vi "Update BrowerTree Component.vi"(6 "SymbolIndex":T1=enum."Project", 8 "error in (no error)":errorcluster, 9 "BrowerComponentNewName(\"\")":string, 10 "BrowerComponentID(\"\")":string, 11 "BrowerTree in":refnum<class "BrowerTree.lvclass">) -> (0 "error out":errorcluster, 3 "BrowerTree out":refnum<class "BrowerTree.lvclass">)   [LabVIEW 2015, in "BrowerTree.lvclass"]
uses:
  BrowerTree.lvclass
  Type Definition/Symbol Index.ctl
  BrowerTree.lvclass/BrowerTree.ctl
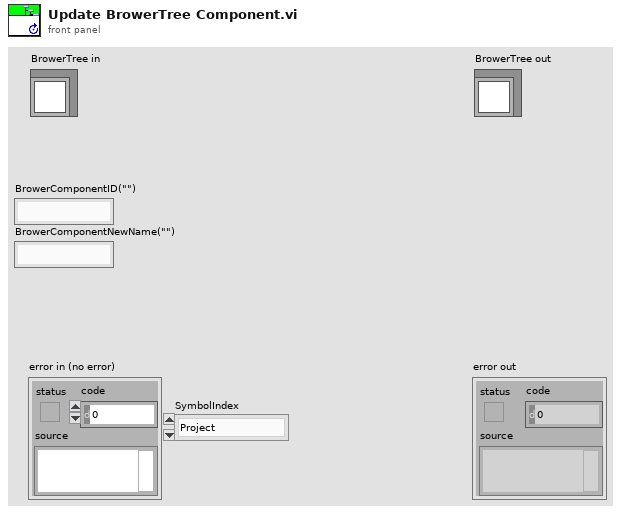
[diagram p1: front panel]
types:
  T1 = typedef "BrowerTree.lvclass/Symbol Index.ctl" = enum16{"PC", "Project", "Module", "DebugTask", "Communication"}
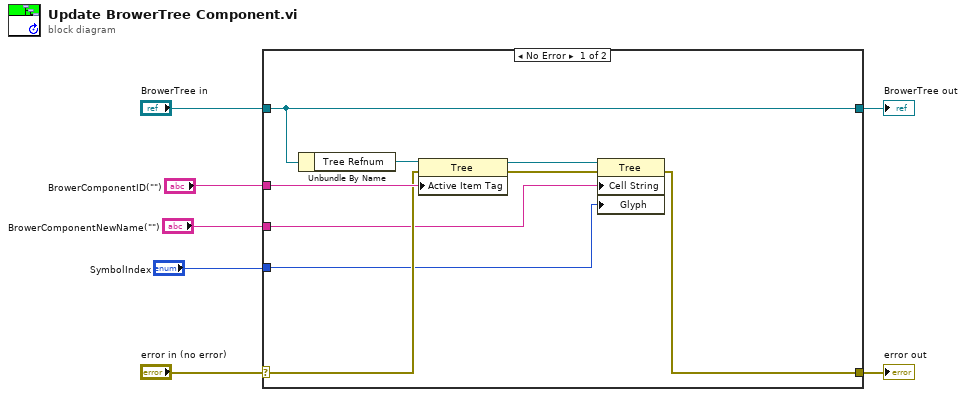
[diagram p0: block diagram]
diagram:
  n1 = case shown="No Error" "error in (no error)" {
    selector: "error in (no error)" -> [w13 w18]
    tunnel: [w8 w18] -> w6
    tunnel: [w16 w17] -> w4
    tunnel: "BrowerTree in" -> [w16 w17]
    tunnel: "BrowerComponentID(\"\")" -> [w14 _]
    tunnel: "BrowerComponentNewName(\"\")" -> [w10 _]
    tunnel: "SymbolIndex" -> [w9 _]
    frame No Error {
      n2 = Unbundle By Name(w16) -> ("Tree Refnum"=w15:refnum<vi>)
      n3 = property class="Tree"(reference=w15, error in=w13, "Active Item Tag"=w14) -> (reference out=w12:refnum<vi>, error out=w11:errorcluster)
      n4 = property class="Tree"(reference=w12, error in=w11, "Cell String"=w10, "Glyph"=w9) -> (error out=w8:errorcluster)  [unwired: 1 out]
    }
    frame Error {
    }
  }
  "error out" <- w6
  "BrowerTree out" <- w4
